vi "test-DiffDriveSim-ALL-TESTS.vi"() -> (3 "All Passed":bool)   [LabVIEW 2019]
panel:
  out "convergence":bool
  out "current":bool
  out "Stability Test":bool
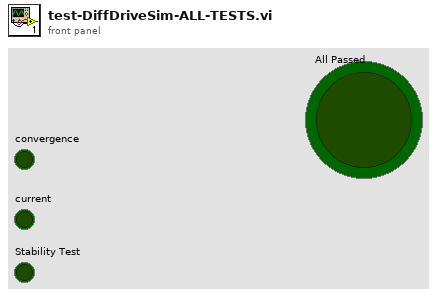
[diagram p1: front panel]
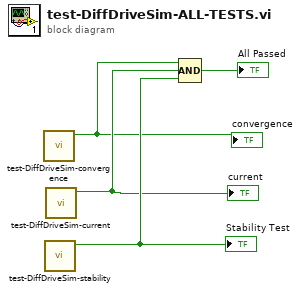
[diagram p0: block diagram]
diagram:
  n1 = call "test-DiffDriveSim-convergence.vi"() -> ("Test Passed"=w1:bool)  [unwired: 11 in]
  "convergence" <- w1
  n2 = call "test-DiffDriveSim-stability.vi"() -> ("Test Passed"=w3:bool)  [unwired: 11 in]
  "Stability Test" <- w3
  n3 = call "test-DiffDriveSim-current.vi"() -> ("Test Passed"=w2:bool)  [unwired: 11 in]
  "current" <- w2
  n4 = Compound Arithmetic op=AND(w1, w2, w3) -> (→"All Passed":bool)
